vi "MakeTextBuffer.vi"(11 "Text":string) -> (2 "size":i32, 3 "Buffer":bool[][](array[boolean]))   [LabVIEW 2020, in "CTI-Peripheral.lvlib" / "Grove I2C Matrix LED Driver.lvclass"]
uses:
  Grove I2C 8x8LEDMatrix/Grove I2C Matrix LED Driver.lvclass
panel:
  # "Input"
  # "Output"
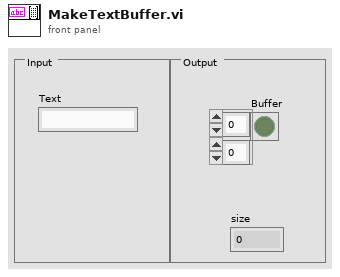
[diagram p1: front panel]
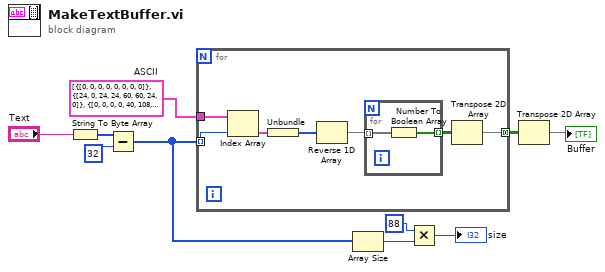
[diagram p0: block diagram]
diagram:
  w4 = cluster{"BytesOut":u8[]}[] [{"BytesOut"=[0, 0, 0, 0, 0, 0, 0, 0]}, {"BytesOut"=[24, 0, 24, 24, 60, 60, 24, 0]}, {"BytesOut"=[0, 0, 0, 0, 40, 108, 108, 0]}, {"BytesOut"=[108, 108, 254, 108, 254, 108, 108, 0]}, {"BytesOut"=[16, 60, 64, 56, 4, 120, 16, 0]}, {"BytesOut"=[96, 102, 12, 24, 48, 102, 6, 0]}, {"BytesOut"=[252, 102, 166, 20, 60, 102, 60, 0]}, {"BytesOut"=[0, 0, 0, 12, 24, 24, 24, 0]}, {"BytesOut"=[96, 48, 24, 24, 24, 48, 96, 0]}, {"BytesOut"=[6, 12, 24, 24, 24, 12, 6, 0]}, {"BytesOut"=[0, 108, 56, 254, 56, 108, 0, 0]}, {"BytesOut"=[0, 16, 16, 124, 16, 16, 0, 0]}, {"BytesOut"=[6, 12, 12, 12, 0, 0, 0, 0]}, {"BytesOut"=[0, 0, 0, 60, 0, 0, 0, 0]}, {"BytesOut"=[6, 6, 0, 0, 0, 0, 0, 0]}, {"BytesOut"=[0, 6, 12, 24, 48, 96, 0, 0]}, {"BytesOut"=[28, 34, 34, 34, 34, 34, 34, 28]}, {"BytesOut"=[28, 8, 8, 8, 8, 8, 12, 8]}, {"BytesOut"=[62, 4, 8, 16, 32, 32, 34, 28]}, {"BytesOut"=[28, 34, 32, 32, 24, 32, 34, 28]}, {"BytesOut"=[32, 32, 62, 34, 36, 40, 48, 32]}, {"BytesOut"=[28, 34, 32, 32, 30, 2, 2, 62]}, {"BytesOut"=[28, 34, 34, 34, 30, 2, 34, 28]}, {"BytesOut"=[4, 4, 4, 8, 16, 32, 32, 62]}, {"BytesOut"=[28, 34, 34, 34, 28, 34, 34, 28]}, {"BytesOut"=[28, 34, 32, 60, 34, 34, 34, 28]}, {"BytesOut"=[0, 24, 24, 0, 24, 24, 0, 0]}, {"BytesOut"=[12, 24, 24, 0, 24, 24, 0, 0]}, {"BytesOut"=[96, 48, 24, 12, 24, 48, 96, 0]}, {"BytesOut"=[0, 0, 60, 0, 60, 0, 0, 0]}, {"BytesOut"=[6, 12, 24, 48, 24, 12, 6, 0]}, {"BytesOut"=[24, 0, 24, 56, 96, 102, 60, 0]}, {"BytesOut"=[0, 60, 66, 26, 58, 34, 28, 0]}, {"BytesOut"=[0, 51, 51, 63, 51, 51, 30, 12]}, {"BytesOut"=[0, 63, 102, 102, 62, 102, 102, 63]}, {"BytesOut"=[0, 60, 102, 3, 3, 3, 102, 60]}, {"BytesOut"=[0, 31, 54, 102, 102, 102, 54, 31]}, {"BytesOut"=[0, 127, 70, 22, 30, 22, 70, 127]}, {"BytesOut"=[0, 15, 6, 22, 30, 22, 70, 127]}, {"BytesOut"=[0, 124, 102, 115, 3, 3, 102, 60]}, {"BytesOut"=[0, 51, 51, 51, 63, 51, 51, 51]}, {"BytesOut"=[0, 30, 12, 12, 12, 12, 12, 30]}, {"BytesOut"=[0, 30, 51, 51, 48, 48, 48, 120]}, {"BytesOut"=[0, 103, 102, 54, 30, 54, 102, 103]}, {"BytesOut"=[0, 127, 102, 70, 6, 6, 6, 15]}, {"BytesOut"=[0, 99, 99, 107, 127, 127, 119, 99]}, {"BytesOut"=[0, 99, 99, 115, 123, 111, 103, 99]}, {"BytesOut"=[0, 28, 54, 99, 99, 99, 54, 28]}, {"BytesOut"=[0, 15, 6, 6, 62, 102, 102, 63]}, {"BytesOut"=[0, 56, 30, 59, 51, 51, 51, 30]}, {"BytesOut"=[0, 103, 102, 54, 62, 102, 102, 63]}, {"BytesOut"=[0, 30, 51, 56, 14, 7, 51, 30]}, {"BytesOut"=[0, 30, 12, 12, 12, 12, 45, 63]}, {"BytesOut"=[0, 63, 51, 51, 51, 51, 51, 51]}, {"BytesOut"=[0, 12, 30, 51, 51, 51, 51, 51]}, {"BytesOut"=[0, 99, 119, 127, 107, 99, 99, 99]}, {"BytesOut"=[0, 99, 54, 28, 28, 54, 99, 99]}, {"BytesOut"=[0, 30, 12, 12, 30, 51, 51, 51]}, {"BytesOut"=[0, 127, 102, 76, 24, 49, 99, 127]}, {"BytesOut"=[120, 24, 24, 24, 24, 24, 120, 0]}, {"BytesOut"=[0, 96, 48, 24, 12, 6, 0, 0]}, {"BytesOut"=[30, 24, 24, 24, 24, 24, 30, 0]}, {"BytesOut"=[0, 0, 0, 130, 68, 40, 16, 0]}, {"BytesOut"=[126, 0, 0, 0, 0, 0, 0, 0]}, {"BytesOut"=[0, 0, 0, 0, 96, 48, 48, 0]}, {"BytesOut"=[0, 110, 51, 62, 48, 30, 0, 0]}, {"BytesOut"=[0, 59, 102, 102, 62, 6, 6, 7]}, {"BytesOut"=[0, 30, 51, 3, 51, 30, 0, 0]}, {"BytesOut"=[0, 110, 51, 51, 62, 48, 48, 56]}, {"BytesOut"=[0, 30, 3, 63, 51, 30, 0, 0]}, {"BytesOut"=[0, 15, 6, 6, 15, 6, 54, 28]}, {"BytesOut"=[31, 48, 62, 51, 51, 110, 0, 0]}, {"BytesOut"=[0, 103, 102, 102, 110, 54, 6, 7]}, {"BytesOut"=[0, 30, 12, 12, 12, 14, 0, 12]}, {"BytesOut"=[30, 51, 51, 48, 48, 48, 0, 48]}, {"BytesOut"=[0, 103, 54, 30, 54, 102, 6, 7]}, {"BytesOut"=[0, 30, 12, 12, 12, 12, 12, 14]}, {"BytesOut"=[0, 99, 107, 127, 127, 51, 0, 0]}, {"BytesOut"=[0, 51, 51, 51, 51, 31, 0, 0]}, {"BytesOut"=[0, 30, 51, 51, 51, 30, 0, 0]}, {"BytesOut"=[15, 6, 62, 102, 102, 59, 0, 0]}, {"BytesOut"=[120, 48, 62, 51, 51, 110, 0, 0]}, {"BytesOut"=[0, 15, 6, 102, 110, 59, 0, 0]}, {"BytesOut"=[0, 31, 48, 30, 3, 62, 0, 0]}, {"BytesOut"=[0, 24, 44, 12, 12, 62, 12, 8]}, {"BytesOut"=[0, 110, 51, 51, 51, 51, 0, 0]}, {"BytesOut"=[0, 12, 30, 51, 51, 51, 0, 0]}, {"BytesOut"=[0, 54, 127, 127, 107, 99, 0, 0]}, {"BytesOut"=[0, 99, 54, 28, 54, 99, 0, 0]}, {"BytesOut"=[31, 48, 62, 51, 51, 51, 0, 0]}, {"BytesOut"=[0, 63, 38, 12, 25, 63, 0, 0]}, {"BytesOut"=[112, 24, 24, 12, 24, 24, 112, 0]}, {"BytesOut"=[0, 8, 8, 8, 8, 8, 8, 0]}, {"BytesOut"=[14, 24, 24, 48, 24, 24, 14, 0]}, {"BytesOut"=[0, 0, 0, 54, 92, 0, 0, 0, 0, 0, 0, 0, 0]}]  # ASCII
  n1 = String To Byte Array(string="Text") -> (unsigned byte array=w2:u8[])
  n2 = Subtract(x=w2, y=32) -> (x-y=w5:i32[])
  n3 = for {
    tunnel: w5 -> [w17] mode=indexing
    tunnel: w4 -> [w16]
    tunnel: [w12] -> w7 mode=concatenating
    n4 = Index Array(array=w16, index=w17) -> (element=w15:cluster{"BytesOut":u8[]})
    n5 = Unbundle(w15) -> ("BytesOut"=w13:u8[])
    n6 = Reverse 1D Array(array=w13) -> (reversed array=w11:u8[])
    n7 = for {
      tunnel: w11 -> [w19] mode=indexing
      tunnel: [w18] -> w14 mode=indexing
      n8 = Number To Boolean Array(number=w19) -> (Boolean array=w18:bool[])
    }
    n9 = Transpose 2D Array(2D array=w14) -> (transposed array=w12:bool[][])
  }
  n10 = Array Size(array=w5) -> (size(s)=w6:i32)
  n11 = Multiply(x=88, y=w6) -> (x*y=→"size":i32)
  n12 = Transpose 2D Array(2D array=w7) -> (transposed array=→"Buffer":bool[][])
